vi "set_amplitude.vi"(8 "error in (no error)":errorcluster, 10 "amplitude in":dbl, 11 "FPGAWrapperMH120124RAPS_PXI7813R in":refnum<class "FPGAWrapperMH120124RAPS_PXI7813R.lvclass">) -> (0 "error out":errorcluster, 3 "FPGAWrapperMH120124RAPS_PXI7813R out":refnum<class "FPGAWrapperMH120124RAPS_PXI7813R.lvclass">)   [LabVIEW 2010, in "FPGAWrapperMH120124RAPS_PXI7813R.lvclass"]
uses:
  FPGAWrapperMH120124RAPS_PXI7813R.lvclass
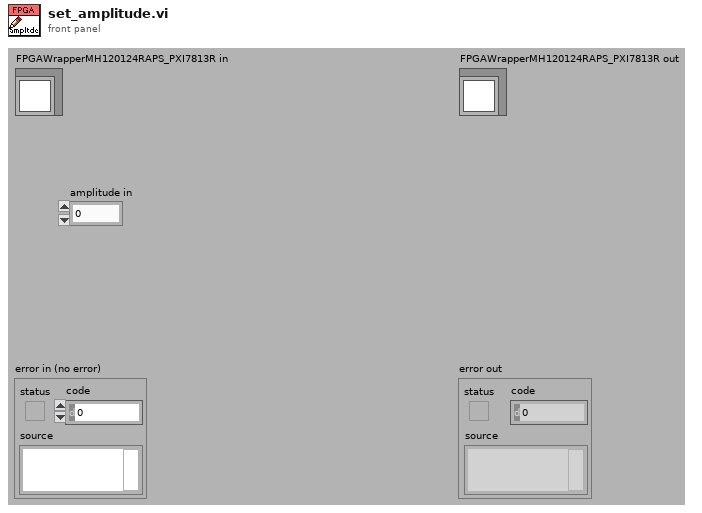
[diagram p1: front panel]
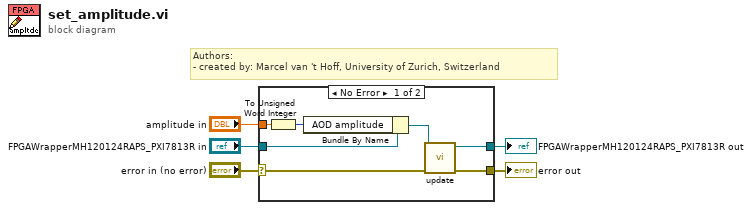
[diagram p0: block diagram]
diagram:
  # "Authors: \n- created by: Marcel van 't Hoff, University of Zurich, Switzerland"
  n1 = case shown="No Error" "error in (no error)" {
    selector: "error in (no error)" -> [w11 w14]
    tunnel: [w7 w14] -> w1
    tunnel: [w8 w13] -> w2
    tunnel: "FPGAWrapperMH120124RAPS_PXI7813R in" -> [w10 w13]
    tunnel: "amplitude in" -> [w12 _]
    frame No Error {
      n2 = To Unsigned Word Integer(number=w12) -> (unsigned 16bit integer=w6:u16)
      n3 = Bundle By Name(cluster=w10, "AOD amplitude"=w6) -> (w9:refnum<class "FPGAWrapperMH120124RAPS_PXI7813R.lvclass">)
      n4 = call-dynamic "update.vi"("error in (no error)"=w11, "FPGAWrapperMH120124RAPS_PXI7813R in"=w9) -> ("error out"=w7:errorcluster, "FPGAWrapperMH120124RAPS_PXI7813R out"=w8:refnum<class "FPGAWrapperMH120124RAPS_PXI7813R.lvclass">)  [unwired: 8 in]
    }
    frame Error {
    }
  }
  "error out" <- w1
  "FPGAWrapperMH120124RAPS_PXI7813R out" <- w2
